vi "Write Nested Viewable Enqueuers.vi"(8 "error in (no error)":errorcluster, 9 "Viewable Names (optional)":string[](array[string]), 10 "Nested Viewable Enqueuers":refnum<class "Message Enqueuer.lvclass">[](array[class]), 11 "IViewManager In":refnum<class "IViewManager.lvclass">) -> (0 "error out":errorcluster, 3 "IViewManager Out":refnum<class "IViewManager.lvclass">)   [LabVIEW 2017, in "IViewManager.lvlib" / "IViewManager.lvclass"]
doc: "<License>\nCopyright © 2017 Composed Systems, LLC | All rights reserved\nwww.composed.io\n\nAuthor: Ethan Stern <ethan.stern@composed.io>\n\nThis software is provided \"AS IS\" WITHOUT WARRANTIES, either express or implied, AND IS FOR EDUCATIONAL PURPOSES ONLY.\n</License>"
uses:
  IViewManager.lvclass
  <vilib>/ActorFramework/Message Enqueuer/Message Enqueuer.lvclass
  IViewManager.lvclass/IViewManager.ctl
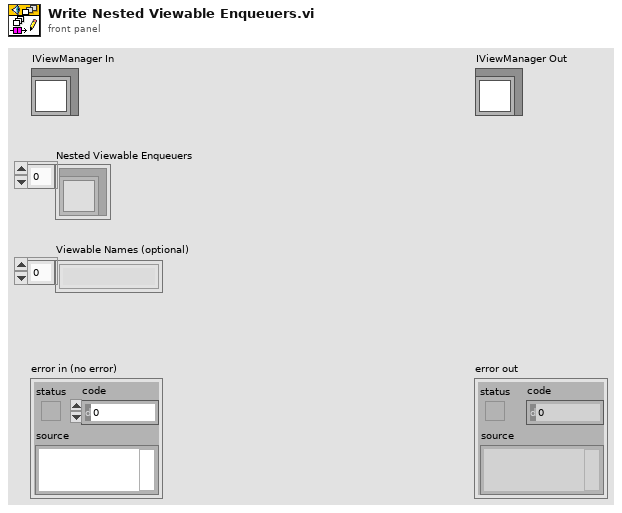
[diagram p1: front panel]
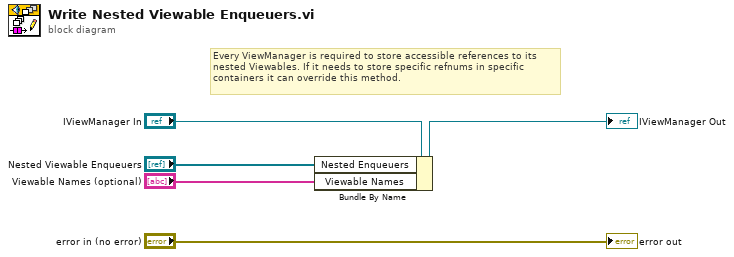
[diagram p0: block diagram]
diagram:
  # "Every ViewManager is required to store accessible references to its\nnested Viewables. If it needs to store specific refnums in specific\ncontainers it can override this method."
  n1 = Bundle By Name(cluster="IViewManager In", "Nested Enqueuers"="Nested Viewable Enqueuers", "Viewable Names"="Viewable Names (optional)") -> (→"IViewManager Out":refnum<class "IViewManager.lvclass">)
  "error out" <- "error in (no error)"
